vi "configAO.vi"(8 "error in (no error)":errorcluster, 10 "address":string, 11 "Channels: AO in":T1 {"AO f (Hz)" min=0.001 max=10000.0; "AO DC (V)" format="%#_6p"; "AO amp (V)" format="%#_6p"}) -> (0 "error out":errorcluster, 3 "Channels: AO out":T1 {"AO f (Hz)" min=0.001 max=10000.0; "AO DC (V)" format="%#_6p"; "AO amp (V)" format="%#_6p"})   [LabVIEW 2016]
uses:
  Typedefs/AO-cluster.ctl
  Typedefs/AO_Amp-array.ctl
  Typedefs/AO_DC-array.ctl
  Typedefs/AO_f-array.ctl
  Typedefs/AO_phi-array.ctl
  Typedefs/Function-array.ctl
  Typedefs/Function-enum.ctl
  RemoteControl/Typedefs/Remote-SMO-Commands-Enum.ctl
  <vilib>/addons/_JKI.lib/Serialization/JSON/JKI JSON Serialization.lvlib
  RemoteControl/RemoteControl.lvclass
panel:
  # "0"
  # "1"
  # "2"
  # "3"
  # "4"
  # "5"
  # "6"
  # "7"
  # "0"
  # "1"
  # "2"
  # "3"
  # "4"
  # "5"
  # "6"
  # "7"
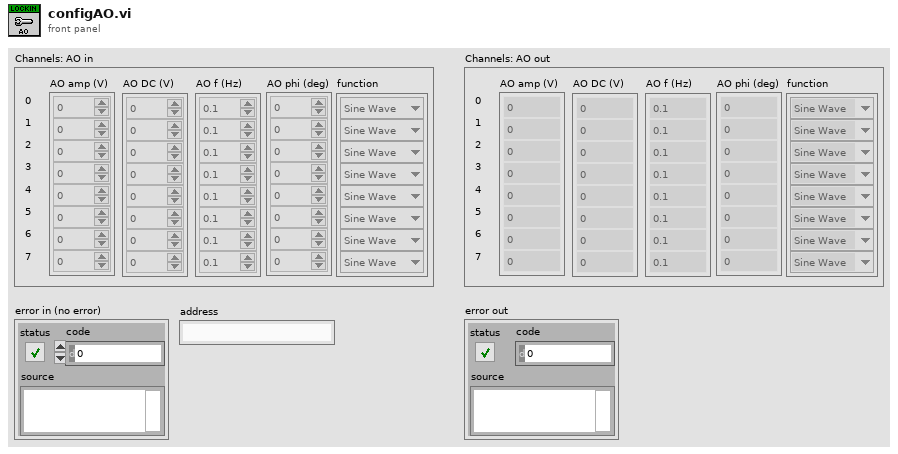
[diagram p1: front panel]
types:
  T1 = typedef "AO-cluster.ctl" = cluster{"AO amp (V)":T2, "AO DC (V)":T3, "AO f (Hz)":T4, "AO phi (deg)":T5, "function":T6}
  T2 = typedef "AO_Amp-array.ctl" = dbl[]
  T3 = typedef "AO_DC-array.ctl" = dbl[]
  T4 = typedef "AO_f-array.ctl" = dbl[]
  T5 = typedef "AO_phi-array.ctl" = dbl[]
  T6 = typedef "Function-array.ctl" = T7[]
  T7 = typedef "Function-enum.ctl" = enum16{"Sine Wave", "Triangle Wave", "Square Wave", "Sawtooth Wave"}
  T8 = typedef "RemoteControl.lvclass/Remote-SMO-Commands-Enum.ctl" = enum16{"configAO", "configREF", "configIVmode", "configRemote", "ACK", "UNK", "CLOSE"}
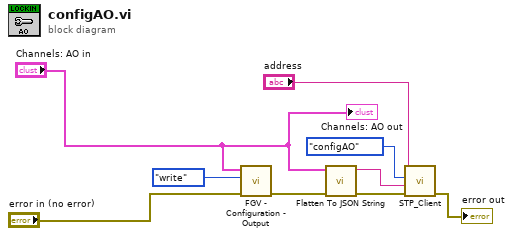
[diagram p0: block diagram]
diagram:
  n1 = call "FGV - Configuration - Output.vi"("error in"="error in (no error)", "Function"=enum16{"write", "read"}."write", "Channels: AO"="Channels: AO in") -> ("error out"=w8:errorcluster)  [unwired: 3 in, 1 out]
  n2 = call <vilib>:"Flatten To JSON String.vi"("error in (no error)"=w8, "Variant"="Channels: AO in") -> ("error out"=w7:errorcluster, "JSON String"=w6:string)  [unwired: 8 in]
  n3 = call "STP_Client.vi"("error in (no error)"=w7, "data to send"=w6, "Command"=Remote-SMO-Commands-Enum."configAO", "address"="address") -> ("error out"=→"error out":errorcluster)  [unwired: 7 in]
  "Channels: AO out" <- "Channels: AO in"
